vi "Stop Server.vi"(0 "WebSocket Server Manager in":refnum<class "WebSocket Server Manager.lvclass">, 2 "Receive Server Enqueuer Handler":refnum<class "WebSocket Server-Service Enqueuer Msg.lvclass">, 5 "Listener Settings":T1={"resolve remote address (T)"=TRUE, "timeout ms (-1)"=-1, "net address"=0, "port"=6163}, 7 "Handshake timeout (5000 ms)":i32=5000, 9 "Subscriber Enqueuer":refnum<class "Message Enqueuer.lvclass">, 11 "error in (no error)":errorcluster) -> (4 "WebSocket Server Manager out":refnum<class "WebSocket Server Manager.lvclass">, 15 "error out":errorcluster)   [LabVIEW 2016, in "WebSocket Actors.lvlib" / "WebSocket Server Manager.lvclass"]
doc: "This method stops a server listening on at a specified port and interface address as detailed in the \"Listener Settings\" input."
uses:
  WebSocket Server Manager.lvclass
  WebSocket Server/typedefs/Listener Settings.ctl
  <vilib>/ActorFramework/Message Enqueuer/Message Enqueuer.lvclass
  Abstract Messages/WebSocket Server-Service Enqueuer Msg/WebSocket Server-Service Enqueuer Msg.lvclass
  C:/Program Files (x86)/National Instruments/LabVIEW 2016/vi.lib/ActorFramework/Message/Message.lvclass
  WebSocket Server Manager.lvclass/WebSocket Server Manager.ctl
  <vilib>/ActorFramework/Message Enqueuer/Message Enqueuer.lvclass/Message Enqueuer.ctl
  Abstract Messages/WebSocket Server-Service Enqueuer Msg/WebSocket Server-Service Enqueuer Msg.lvclass/WebSocket Server-Service Enqueuer Msg.ctl
  <vilib>/ActorFramework/Message Enqueuer/Enqueue.vi
  <vilib>/ActorFramework/Stop Msg/Stop Msg.lvclass
  <vilib>/ActorFramework/Message Priority Queue/Priority Enqueue.vi
  <vilib>/Utility/error.llb/Error Cluster From Error Code.vi
  <vilib>/ErrorRing/Error Ring.xnode
  WebSocket Server/WebSocket Server.lvclass
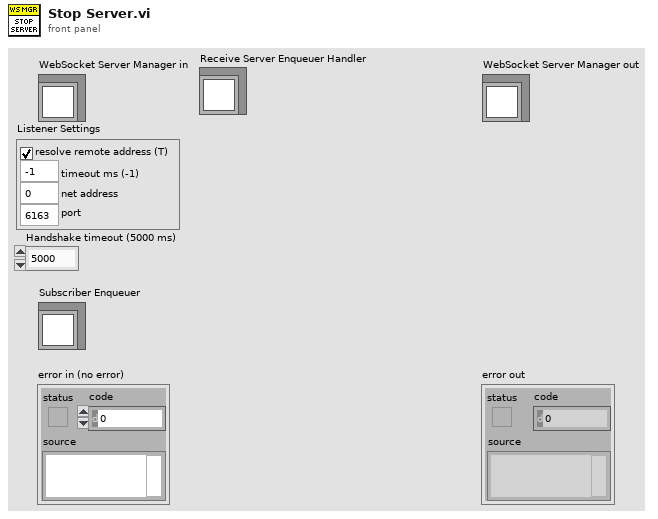
[diagram p1: front panel]
types:
  T1 = typedef "WebSocket Actors.lvlib/WebSocket Server.lvclass/Listener Settings.ctl" = cluster{"resolve remote address (T)":bool, "timeout ms (-1)":i32, "net address":u32, "port":u16}
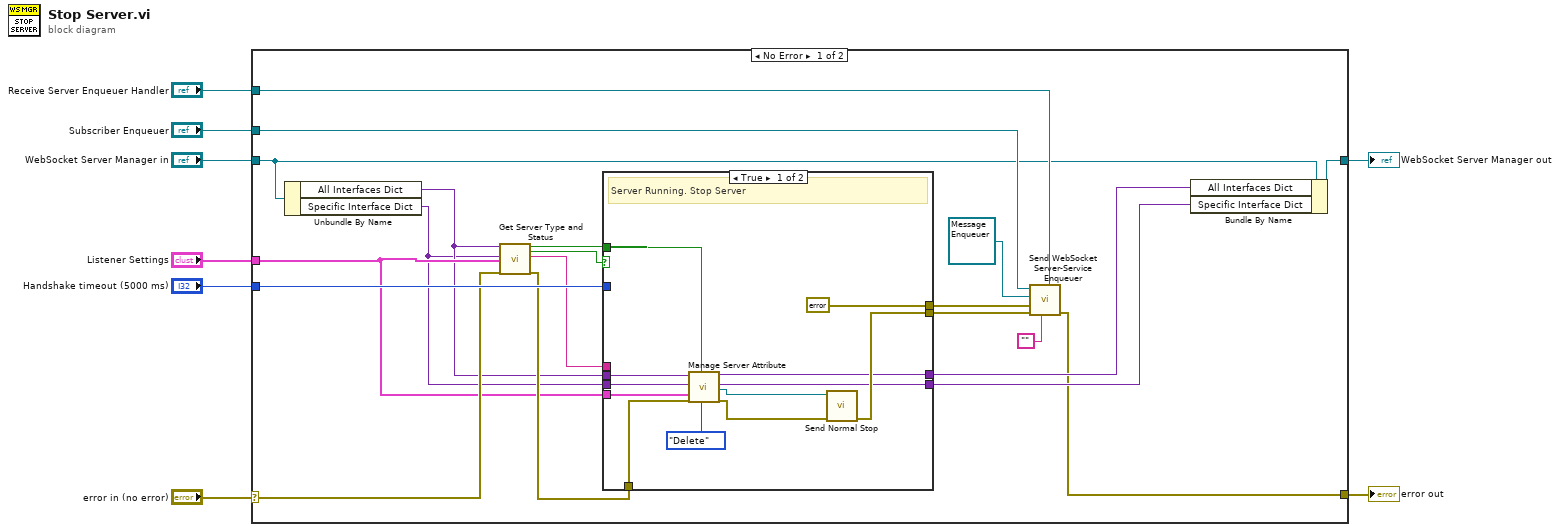
[diagram p0: block diagram]
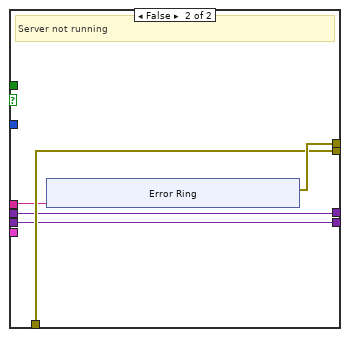
[diagram p2: hidden frame]
diagram:
  n1 = case shown="No Error" "error in (no error)" {
    selector: "error in (no error)" -> [w26 w54]
    tunnel: [w18 w54] -> w7
    tunnel: [w28 w53] -> w5
    tunnel: "WebSocket Server Manager in" -> [w11 w53]
    tunnel: "Handshake timeout (5000 ms)" -> [w27 _]
    tunnel: "Listener Settings" -> [w14 _]
    tunnel: "Subscriber Enqueuer" -> [w23 _]
    tunnel: "Receive Server Enqueuer Handler" -> [w17 _]
    frame No Error {
      n2 = Unbundle By Name(w11) -> ("All Interfaces Dict"=w13:variant, "Specific Interface Dict"=w12:variant)
      n3 = call "Get Server Type and Status.vi"("All Interfaces Dict"=w13, "Specific Interface Dict in"=w12, "Listener Settings"=w14, "error in (no error)"=w26) -> ("Is \"All Interface\" Server"=w21:bool, "Server Running"=w25:bool, "Server URI"=w16:string, "error out"=w15:errorcluster)  [unwired: 12 in]
      n4 = case shown="True" w25 {
        tunnel: w27 -> [_ _]
        tunnel: w14 -> [w30 _]
        tunnel: w15 -> [w40 w44]
        tunnel: w16 -> [_ w41]
        tunnel: [w35 w44] -> w24
        tunnel: [errorcluster {"status"=FALSE, "code"=0, "source"=""} ("error out") w45] -> w22
        tunnel: w21 -> [w29 _]
        tunnel: w13 -> [w37 w43]
        tunnel: [w33 w42] -> w20
        tunnel: [w32 w43] -> w19
        tunnel: w12 -> [w36 w42]
        frame True {
          # "Server Running. Stop Server"
          n5 = call "Manage Server Attribute.vi"("All Interfaces Dict in"=w37, "Specific Interface Dict in"=w36, "Listener Settings"=w30, "error in (no error)"=w40, "Is \"All Interface\" Server"=w29, "Action"=enum16{"Set", "Get", "Delete"}."Delete") -> ("All Interfaces Dict out"=w32:variant, "Specific Interface Dict out"=w33:variant, "Message Enqueuer out"=w34:refnum<class "Message Enqueuer.lvclass">, "error out"=w31:errorcluster)  [unwired: 10 in]
          n6 = call <vilib>:"Send Normal Stop.vi"("error in (no error)"=w31, "Message Enqueuer"=w34) -> ("error out"=w35:errorcluster)  [unwired: 9 in]
        }
        frame False {
          # "Server not running"
          n7 = xnode "Error Ring"("parameter 0"=w41) -> ("error out"=w45:errorcluster)
        }
      }
      n8 = call "Send WebSocket Server-Service Enqueuer.vi"("Receive Service/Server Enqueuer Handler"=w17, "Service Name"="", "error in (no error)"=w24, "Error"=w22, "WebSocket Server/Service Enqueuer"=refnum<class "Message Enqueuer.lvclass"> refnum ("Message Enqueuer"), "Message Enqueuer"=w23) -> ("error out"=w18:errorcluster)  [unwired: 4 in, 1 out]
      n9 = Bundle By Name(cluster=w11, "All Interfaces Dict"=w19, "Specific Interface Dict"=w20) -> (w28:refnum<class "WebSocket Server Manager.lvclass">)
    }
    frame Error {
    }
  }
  "error out" <- w7
  "WebSocket Server Manager out" <- w5
